vi "example_03_three_button.vi"() -> ()   [LabVIEW 2015, in "lv-dialog.lvlib" / "v1.lvlib"]
uses:
  v1.lvlib
  public/_controls/dialog_selection.ctl
  public/class/v1.lvclass
panel:
  in  "boolean_text_3":string="Cancel"
  in  "boolean_text_2":string="No"
  in  "boolean_text_1":string="Yes"
  in  "dialog_text":string="Press a button"
  out "error":errorcluster
  out "dialog_selection":T1
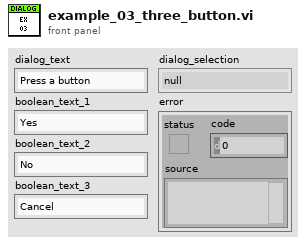
[diagram p1: front panel]
types:
  T1 = typedef "lv-dialog.lvlib/v1.lvlib/dialog_selection.ctl" = enum16{"null", "panel_closed", "button_1", "button_2", "button_3", "cancelled"}
  T2 = cluster{"dialog_text":string, "boolean_text_1":string, "boolean_text_2":string, "boolean_text_3":string}
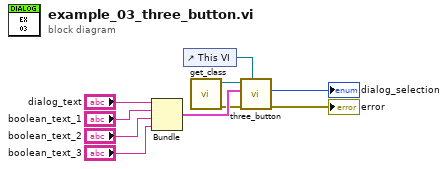
[diagram p0: block diagram]
diagram:
  n1 = Bundle("dialog_text"="dialog_text", "boolean_text_1"="boolean_text_1", "boolean_text_2"="boolean_text_2", "boolean_text_3"="boolean_text_3") -> (w5:T2)  [unwired: 1 in]
  n2 = control-ref of="This VI"() -> (w10:refnum<vi>)
  n3 = call "get_class.vi"() -> ("error out"=w3:errorcluster, "class"=w4:refnum<class "v1.lvclass">)  [unwired: 10 in]
  n4 = call-dynamic "three_button.vi"("callee"=w10, "error in (no error)"=w3, "configuration"=w5, "v1 in"=w4) -> ("error out"=→"error":errorcluster, "dialog_selection"=→"dialog_selection":T1)  [unwired: 5 in, 1 out]
